vi "改变局部变量的数据流方向.vi"() -> ()   [LabVIEW 2010]
panel:
  out "温度显示":dbl
  in  "温度":dbl
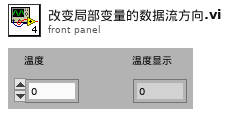
[diagram p1: front panel]
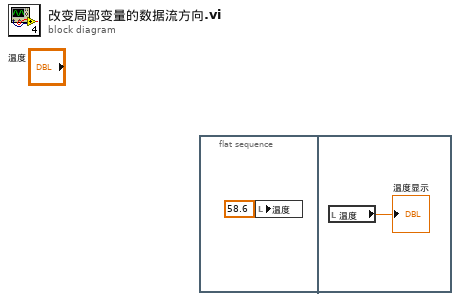
[diagram p0: block diagram]
diagram:
  n1 = flat-sequence {
    frame #0 {
      n2 = local write "温度"(58.6 ("温度")) -> ()
    }
    frame #1 {
      n3 = local read "温度"() -> (→"温度显示":dbl)
    }
  }
